vi "Ramp Voltage Keithley 2450.vi"() -> ()   [LabVIEW 2020]
panel:
  out "Voltage":dbl format="%.6g"
  in  "stop":bool
  in  "Dwell (S)":dbl=1.0 format="%.5g"
  out "String":string
  in  "Step Size":dbl=0.0003 format="%.5g"
  in  "End Voltage":dbl=10.0 format="%.5g"
  in  "Start Voltage":dbl=-10.0 format="%.5g"
  in  "VISA resource name":refnum<visa-resource-name>="tcpip::k-2450-00000000.ad.magnet.fsu.edu::INSTR"
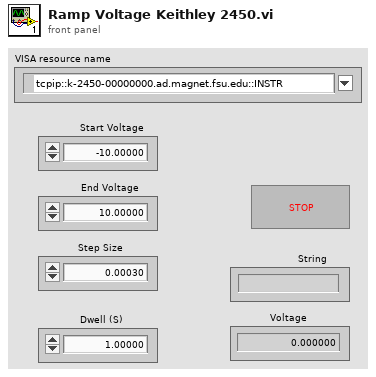
[diagram p1: front panel]
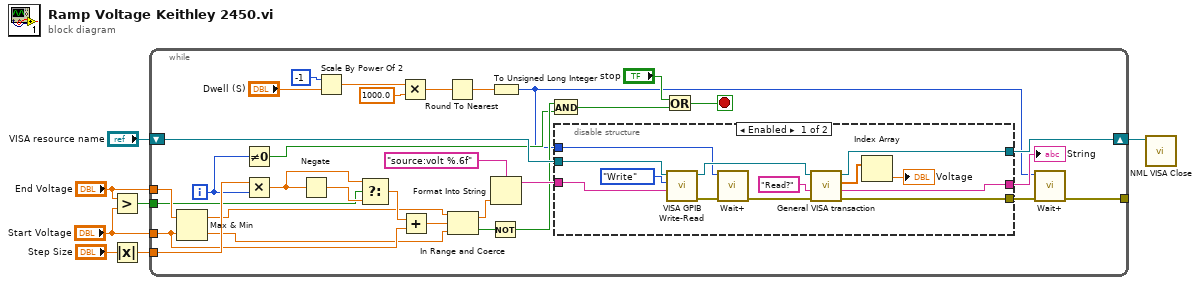
[diagram p0: block diagram]
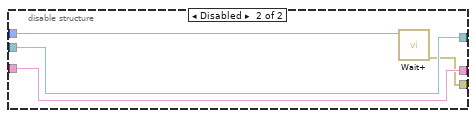
[diagram p2: hidden frame]
diagram:
  n1 = Greater?(x="End Voltage", y="Start Voltage") -> (0:w4:bool)
  n2 = Absolute Value(x="Step Size") -> (abs(x)=w1:dbl)
  n3 = while {
    shift-right: [w38] -> w6
    shift-left: "VISA resource name" -> [w39]
    tunnel: w1 -> [w35]
    tunnel: w4 -> [w30]
    tunnel: "Start Voltage" -> [w20]
    tunnel: "End Voltage" -> [w31]
    tunnel: [w28] -> _
    i -> [w16]
    stop <- w24 stop-if-true
    n4 = Max & Min(x=w31, y=w20) -> (max(x,y)=w18:dbl, min(x,y)=w19:dbl)
    n5 = Not Equal To 0?(x=w16) -> (x != 0?=w14:bool)
    n6 = Multiply(x=w35, y=w16) -> (x*y=w33:dbl)
    n7 = Negate(x=w33) -> (-x=w34:dbl)
    n8 = Scale By Power Of 2(n=i16 -1, x="Dwell (S)") -> (x*2^n=w12:dbl)
    n9 = Select(t=w33, s=w30, f=w34) -> (s? t:f=w32:dbl)
    n10 = Multiply(x=w12, y=1000.0) -> (x*y=w10:dbl)
    n11 = Add(x=w32, y=w20) -> (x+y=w21:dbl)
    n12 = Round To Nearest(number=w10) -> (nearest integer value=w8:dbl)
    n13 = In Range and Coerce(upper limit=w18, x=w21, lower limit=w19) -> (coerced(x)=w22:dbl, In Range?=w23:bool)
    n14 = Not(x=w23) -> (.not. x?=w17:bool)
    n15 = To Unsigned Long Integer(number=w8) -> (unsigned 32bit integer=w9:u32)
    n16 = Format Into String(format string="source:volt %.6f", w22) -> (resulting string=w37:string)  [unwired: 2 in, 1 out]
    n17 = And(x=w17, y=w14) -> (x .and. y?=w15:bool)
    n18 = disable-structure shown="Enabled" {
      disable-tunnel: w39 -> [w51 w56]
      disable-tunnel: [w50 w56] -> w38
      disable-tunnel: w37 -> [w48 w55]
      disable-tunnel: [w45 w53] -> w29
      disable-tunnel: [w42 w55] -> w13
      disable-tunnel: w9 -> [w40 w54]
      frame Enabled {
        n19 = call "VISA GPIB Write-Read.vi"("Command"=w48, "Action"=enum16{"Write", "Read", "Write & Read"}."Write", "VISA resource name"=w51) -> ("error out"=w46:errorcluster, "dup VISA Session"=w52:refnum<visa-resource-name>)  [unwired: 5 in, 2 out]
        n20 = call "Wait+.vi"("Error In"=w46, "milliseconds to wait"=w40) -> ("Error Out"=w41:errorcluster)  [unwired: 4 in, 1 out]
        n21 = call "General VISA transaction.vi"("error in (no error)"=w41, "Command String"="Read?", "VISA Session"=w52) -> ("error out"=w45:errorcluster, "String Resonse"=w42:string, "Measurement"=w44:dbl[], "dup VISA Session"=w50:refnum<visa-resource-name>)  [unwired: 3 in, 2 out]
        n22 = Index Array(array=w44) -> (element=→"Voltage":dbl)  [unwired: 1 in]
      }
      frame Disabled {
        n23 = call "Wait+.vi"("milliseconds to wait"=w54) -> ("Error Out"=w53:errorcluster)  [unwired: 5 in, 1 out]
      }
    }
    "String" <- w13
    n24 = Or(x="stop", y=w15) -> (x .or. y?=w24:bool)
    n25 = call "Wait+.vi"("Error In"=w29, "milliseconds to wait"=w9) -> ("Error Out"=w28:errorcluster)  [unwired: 4 in, 1 out]
  }
  n26 = call "NML VISA Close.vi"("VISA resource name"=w6) -> ()  [unwired: 10 in, 1 out]
